vi "MTIF_Create.vi"(5 "Byte Order":T1(ring)=enum."little-endian", 6 "Bytes per pixel":u8=1, 7 "ROI Rectangle":i32[](array[numeric]), 8 "error in (no error)":errorcluster, 9 "Frame Rate (fps)":dbl, 10 "File Name (.mtif)":string="zebrafish_2", 11 "Folder Path":path=path "X:/Zebrafish_IR_08_11_2017") -> (0 "error out":errorcluster, 3 "Byte Stream File out":refnum<file>)   [LabVIEW 2019]
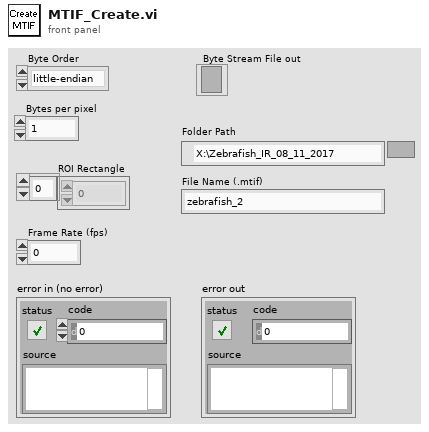
[diagram p1: front panel]
types:
  T1 = enum16{"big-endian, network order", "native, host order", "little-endian"}
  T2 = enum16{"deny read/write", "deny write-only", "deny none"}
  T3 = enum16{"open", "replace", "create", "open or create", "replace or create", "replace or create with confirmation"}
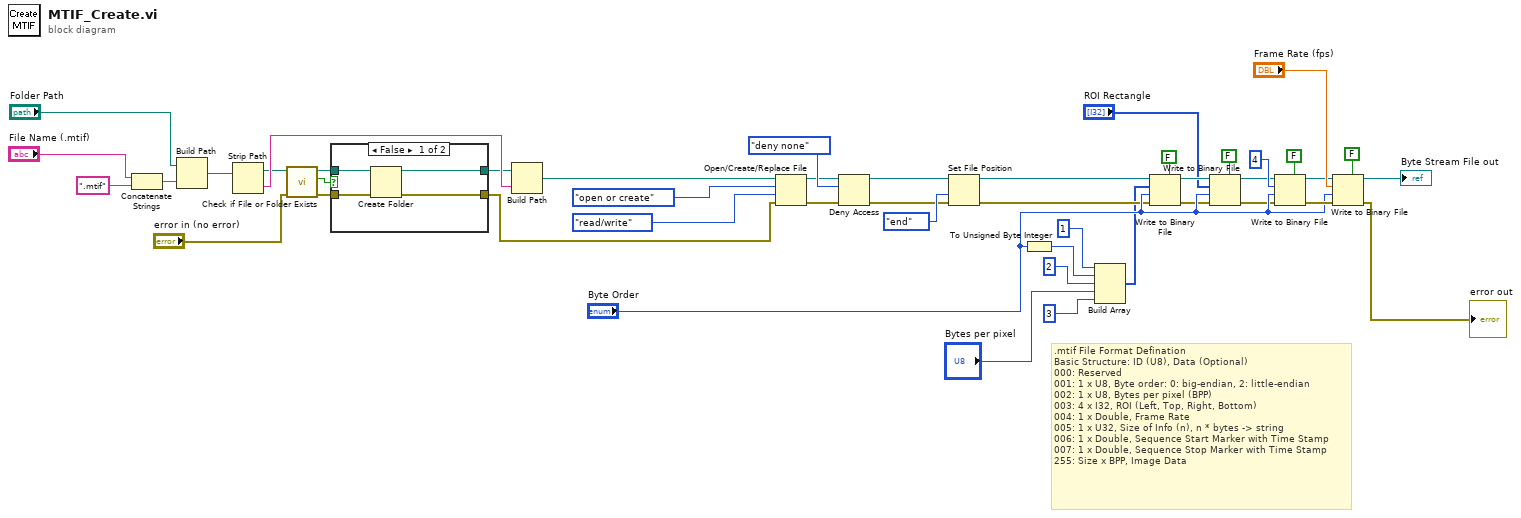
[diagram p0: block diagram]
diagram:
  # ".mtif File Format Defination\nBasic Structure: ID (U8), Data (Optional)\n000: Reserved\n001: 1 x U8, Byte order: 0: big-endian, 2: little-endian\n002: 1 x U8, Bytes per pixel (BPP)\n003: 4 x I32, ROI (Left, Top, Right, Bottom)\n004: 1 x Double, Frame Rate\n005: 1 x U32, Size of Info (n), n * bytes -> string\n006: 1 x Double, Sequence Start Marker with Time Stamp\n007: 1 x Double, Sequence Stop Marker with Time Stamp\n255: Size x BPP, Image Data"
  n1 = Concatenate Strings("File Name (.mtif)", ".mtif" ("string")) -> (w4:string)
  n2 = Build Path(base path="Folder Path", name or relative path=w4) -> (appended path=w6:path)
  n3 = Strip Path(path=w6) -> (stripped path=w7:path, name=w12:string)
  n4 = call <vilib>:"Check if File or Folder Exists.vi"("error in (no error)"="error in (no error)", "path"=w7) -> ("error out"=w10:errorcluster, "file or folder exists?"=w8:bool, "dup path"=w9:path)  [unwired: 7 in]
  n5 = case shown="False" w8 {
    tunnel: w9 -> [w50 w52]
    tunnel: w10 -> [w49 w51]
    tunnel: [w48 w52] -> w11
    tunnel: [w47 w51] -> w1
    frame False {
      n6 = Create Folder(path (use dialog)=w50, error in=w49) -> (created path=w48:path, error out=w47:errorcluster)  [unwired: 1 in, 1 out]
    }
    frame True {
    }
  }
  n7 = Build Path(base path=w11, name or relative path=w12) -> (appended path=w2:path)
  n8 = Open/Create/Replace File(file path (use dialog)=w2, error in=w1, operation (0:open)=T3."open or create", access (0:read/write)=enum16{"read/write", "read-only", "write-only"}."read/write") -> (refnum out=w18:refnum<file>, error out=w17:errorcluster)  [unwired: 2 in, 1 out]
  n9 = Deny Access(4:w17, 6:T2."deny none" ("deny mode (0:deny read/write)"), 7:w18) -> (0:w15:errorcluster, 3:w16:refnum<file>)
  n10 = Set File Position(refnum=w16, from (0:start)=enum16{"start", "end", "current"}."end", error in=w15) -> (refnum out=w29:refnum<file>, error out=w30:errorcluster)  [unwired: 1 in]
  n11 = To Unsigned Byte Integer(number="Byte Order") -> (unsigned 8bit integer=w24:u8)
  n12 = Build Array(u8 1, w24, u8 2 ("element"), "Bytes per pixel", u8 3 ("element")) -> (w27:u8[])
  n13 = Write to Binary File(file (use dialog)=w29, data=w27, error in=w30, 5:FALSE ("prepend array or string size? (T)"), 9:"Byte Order") -> (refnum out=w34:refnum<file>, error out=w35:errorcluster)  [unwired: 1 in, 1 out]
  n14 = Write to Binary File(file (use dialog)=w34, data="ROI Rectangle", error in=w35, 5:FALSE ("prepend array or string size? (T)"), 9:"Byte Order") -> (refnum out=w39:refnum<file>, error out=w40:errorcluster)  [unwired: 1 in, 1 out]
  n15 = Write to Binary File(file (use dialog)=w39, data=u8 4, error in=w40, 5:FALSE ("prepend array or string size? (T)"), 9:"Byte Order") -> (refnum out=w44:refnum<file>, error out=w43:errorcluster)  [unwired: 1 in, 1 out]
  n16 = Write to Binary File(file (use dialog)=w44, data="Frame Rate (fps)", error in=w43, 5:FALSE ("prepend array or string size? (T)"), 9:"Byte Order") -> (refnum out=→"Byte Stream File out":refnum<file>, error out=→"error out":errorcluster)  [unwired: 1 in, 1 out]
